vi "Finish Sending.vi"(10 "error in (no error)":errorcluster, 11 "RequestTraceLog in":refnum<class "RequestTraceLog.lvclass">) -> (2 "error out":errorcluster, 3 "RequestTraceLog out":refnum<class "RequestTraceLog.lvclass">)   [LabVIEW 2020, in "HTTP Server.lvlib" / "RequestTraceLog.lvclass"]
uses:
  RequestTraceLog.lvclass
  RequestTraceLog.lvclass/RequestTraceLog.ctl
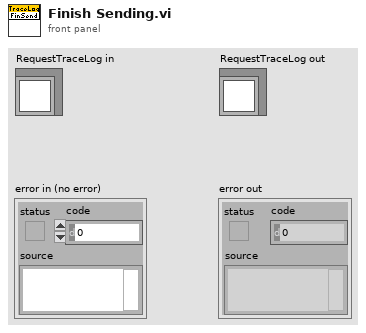
[diagram p1: front panel]
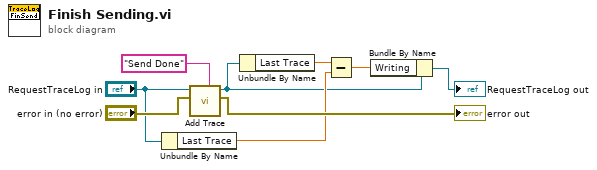
[diagram p0: block diagram]
diagram:
  n1 = Unbundle By Name("RequestTraceLog in") -> ("Last Trace"=w4:dbl)
  n2 = call "Add Trace.vi"("Info"="Send Done", "error in (no error)"="error in (no error)", "RequestTraceLog in"="RequestTraceLog in") -> ("error out"=→"error out":errorcluster, "RequestTraceLog out"=w3:refnum<class "RequestTraceLog.lvclass">)  [unwired: 7 in]
  n3 = Unbundle By Name(w3) -> ("Last Trace"=w5:dbl)
  n4 = Subtract(x=w5, y=w4) -> (x-y=w2:dbl)
  n5 = Bundle By Name(cluster=w3, "Writing"=w2) -> (→"RequestTraceLog out":refnum<class "RequestTraceLog.lvclass">)
